vi "readTEDS.vi"(8 "error in (no error)":errorcluster, 11 "ILC in":refnum<class "ILC.lvclass">) -> (0 "error out":errorcluster, 2 "TEDS Memory":T1, 3 "ILC out":refnum<class "ILC.lvclass">)   [LabVIEW 2015, in "ILCCommon.lvlib" / "ILC.lvclass"]
uses:
  <userlib>/Common/ILC/ILC/ILC.lvclass
  <userlib>/Common/ILC/Typedefs/TEDSMemory.ctl
  <userlib>/Common/ILC/ILCModelTypedefs/FinalDelimiter.ctl
  <userlib>/Common/ILC/ILC/ILC.lvclass/ILC.ctl
  <userlib>/Common/SerialProtocols/SerialCommunicator/SerialCommunicator.lvclass
  <userlib>/Common/ILC/ILCModelTypedefs/ILCModelTypedefs.lvlib
  <userlib>/Common/ILC/Typedefs/ILCTypedefs.lvlib
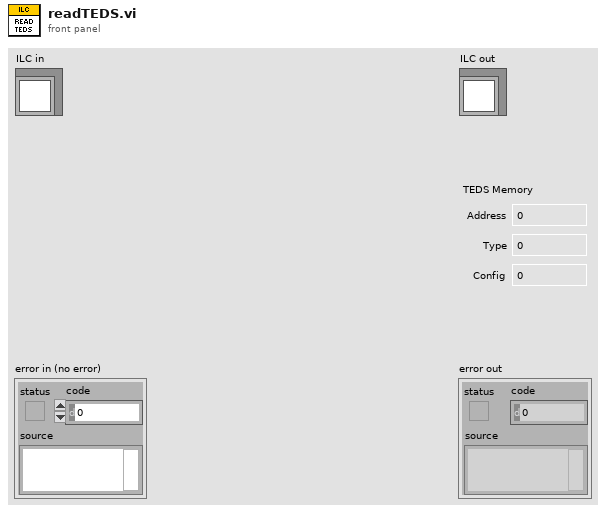
[diagram p1: front panel]
types:
  T1 = typedef "ILCCommon.lvlib/ILCTypedefs.lvlib/TEDSMemory.ctl" = cluster{"Address":i32, "Type":i32, "Config":i32}
  T2 = typedef "ILCCommon.lvlib/ILCModelTypedefs.lvlib/FinalDelimiter.ctl" = enum16{",", "<CR><LF>"}
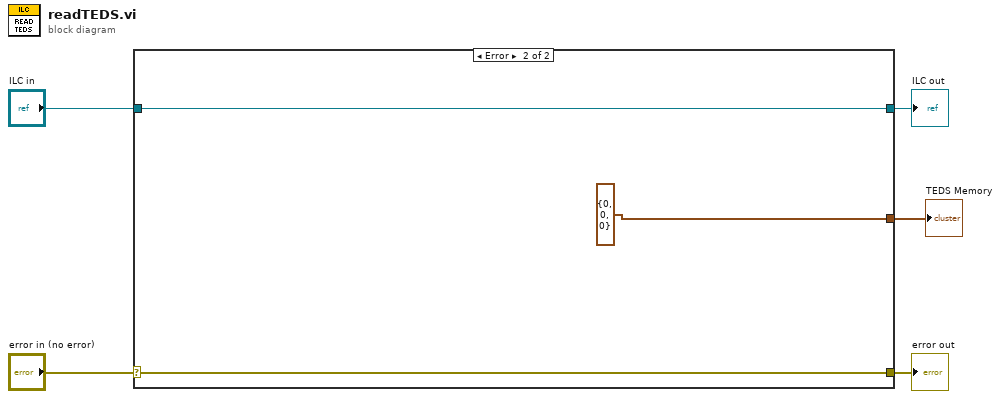
[diagram p0: block diagram]
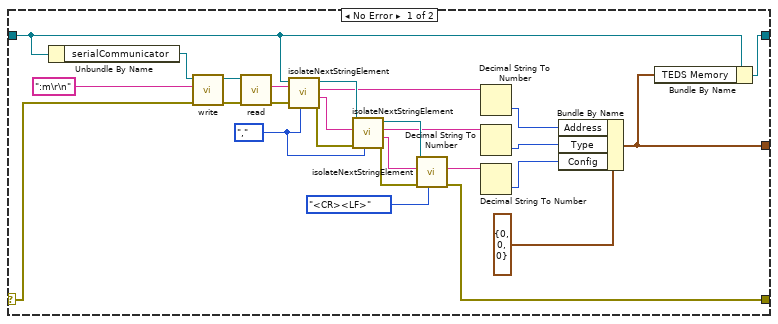
[diagram p2: hidden frame]
diagram:
  n1 = case shown="Error" "error in (no error)" {
    selector: "error in (no error)" -> [w27 w34]
    tunnel: [w10 w34] -> w4
    tunnel: [w8 w33] -> w2
    tunnel: "ILC in" -> [w9 w33]
    tunnel: [w7 T1 {"Address"=0, "Type"=0, "Config"=0} ("TEDS Memory")] -> w1
    frame No Error {
      w17 = FinalDelimiter."," ("Final Delimiter")
      n2 = Unbundle By Name(w9) -> ("serialCommunicator"=w31:refnum<class "SerialCommunicator.lvclass">)
      n3 = call-dynamic "write.vi"("error in (no error)"=w27, "writeString"=":m\r\n", "SerialCommunicator in"=w31) -> ("error out"=w28:errorcluster, "SerialCommunicator out"=w29:refnum<class "SerialCommunicator.lvclass">)  [unwired: 7 in]
      n4 = call-dynamic "read.vi"("error in (no error)"=w28, "SerialCommunicator in"=w29) -> ("error out"=w26:errorcluster, "stringRead"=w25:string)  [unwired: 7 in, 1 out]
      n5 = call <userlib>:"isolateNextStringElement.vi"("Final Delimiter"=w17, "error in (no error)"=w26, "inputString"=w25, "ILC in"=w9) -> ("error out"=w21:errorcluster, "remainingString"=w23:string, "extractedSegment"=w22:string, "ILC out"=w24:refnum<class "ILC.lvclass">)  [unwired: 4 in]
      n6 = call <userlib>:"isolateNextStringElement.vi"("Final Delimiter"=w17, "error in (no error)"=w21, "inputString"=w23, "ILC in"=w24) -> ("error out"=w18:errorcluster, "remainingString"=w19:string, "extractedSegment"=w16:string, "ILC out"=w20:refnum<class "ILC.lvclass">)  [unwired: 4 in]
      n7 = call <userlib>:"isolateNextStringElement.vi"("Final Delimiter"=FinalDelimiter."<CR><LF>", "error in (no error)"=w18, "inputString"=w19, "ILC in"=w20) -> ("error out"=w10:errorcluster, "extractedSegment"=w15:string)  [unwired: 4 in, 2 out]
      n8 = Decimal String To Number(string=w22) -> (number=w13:i32)  [unwired: 2 in, 1 out]
      n9 = Decimal String To Number(string=w16) -> (number=w12:i32)  [unwired: 2 in, 1 out]
      n10 = Decimal String To Number(string=w15) -> (number=w11:i32)  [unwired: 2 in, 1 out]
      n11 = Bundle By Name(cluster=T1 {"Address"=0, "Type"=0, "Config"=0} ("TEDS Memory"), "Address"=w13, "Type"=w12, "Config"=w11) -> (w7:T1)
      n12 = Bundle By Name(cluster=w9, "TEDS Memory"=w7) -> (w8:refnum<class "ILC.lvclass">)
    }
    frame Error {
    }
  }
  "error out" <- w4
  "ILC out" <- w2
  "TEDS Memory" <- w1
